vi "Cursor - Move and Click.vi"(3 "Cursor Position - Write":i32[](array[numeric])) -> ()   [LabVIEW 2013]
uses:
  USER32.DLL
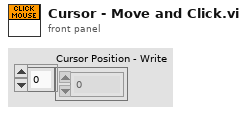
[diagram p1: front panel]
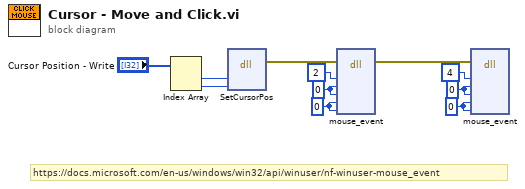
[diagram p0: block diagram]
diagram:
  w8 = 0 ("dwExtraInfo")
  w9 = u32 0 ("dwExtraInfo")
  w6 = 0 ("dwExtraInfo")
  w5 = u32 0 ("dwExtraInfo")
  # "https://docs.microsoft.com/en-us/windows/win32/api/winuser/nf-winuser-mouse_event"
  n1 = Index Array(array="Cursor Position - Write") -> (element #1=w2:i32, element #2=w1:i32)  [unwired: 2 in]
  n2 = dll-call lib="user32.dll" fn="SetCursorPos" label="Move Cursor"("dx"=w2, "dy"=w1) -> (error out=w7:errorcluster)  [unwired: 6 in, 1 out]
  n3 = dll-call lib="user32.dll" fn="mouse_event" label="Left Click - Down"(error in=w7, "dwFlags"=2, "dx"=w6, "dy"=w6, "dwData"=w5, "dwExtraInfo"=w5) -> (error out=w11:errorcluster)  [unwired: 8 in, 1 out]
  n4 = dll-call lib="user32.dll" fn="mouse_event" label="Left Click - Up"(error in=w11, "dwFlags"=4, "dx"=w8, "dy"=w8, "dwData"=w9, "dwExtraInfo"=w9) -> ()  [unwired: 8 in, 2 out]
